vi "getData_v4.vi"() -> ()   [LabVIEW 2014]
uses:
  <vilib>/FPGAPlugInAG/cRIO-9039/niLvFpga_Open_cRIO-9039.vi
  <vilib>/Utility/error.llb/Error Cluster From Error Code.vi
  <vilib>/rvi/errors/niLvFpgaAdjustHostInterfaceError.vi
  <vilib>/Utility/file.llb/Write To Spreadsheet File (DBL).vi
  <vilib>/FPGAPlugInAG/cRIO-9039/niLvFpga_Close_cRIO-9039.vi
  <vilib>/rvi/interface/nirviOpenFPGA/nirviOpenFPGA.xnode
  FPGA Bitfiles/test0304_FPGATarget_imptestv12p4_nHMFqqsr4pc.lvbitx
  FPGA VIs/imp_test_v12_p4.vi
  <vilib>/rvi/interface/nirviMethod/nirviMethod.xnode
  <vilib>/rvi/interface/nirviCloseFPGA/nirviCloseFPGA.xnode
  <vilib>/FPGAPlugInAG/cRIO-9039/niLvFpga_ReadFifo_cRIO-9039.vi
  <vilib>/rvi/errors/niLvFpgaMergeErrorWithErrorCode.vi
panel:
  out "Timer (Sec)":u32
  out "FIFO empty":bool
  out "Elements Remaining":u32=10000
  in  "Time_read":i32=10000
  out "message":string=" INSTRUCTIONS:\r\rNormal Use:  When using subVIs that incorporate the error in/error out (or error I/O) structure, place this handler where you want to inform the user of an error, typically at the end of the I/O data path, as the last action of the program.  If the error in error? is ERROR, the handler creates a message describing the error and its source.  If the type of dialog = 1 (default), the message is displayed to the user, who can only acknowedge it.  If the type = 2, the user can acknowledge the message or abort execution; aborting a program with active I/O is not recommended.  If the type = 0, no message is displayed; this is used to process the error programmatically, and the error out cluster elements are wired to individual terminals for that reason.  \r\rOther Use:\n\r\nlocal testing.  To test the error code of a subVI or function that does not have the error I/O structure, you can wire its error code and a source string to the local error code and error source inputs.  If error in error? indicates no error and error code is not equal to 0, the local code and source are substituted for the error in values, and error? is set TRUE (ERROR)."
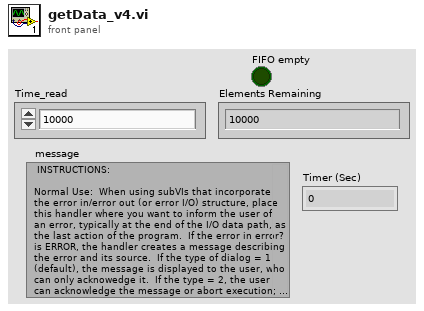
[diagram p1: front panel]
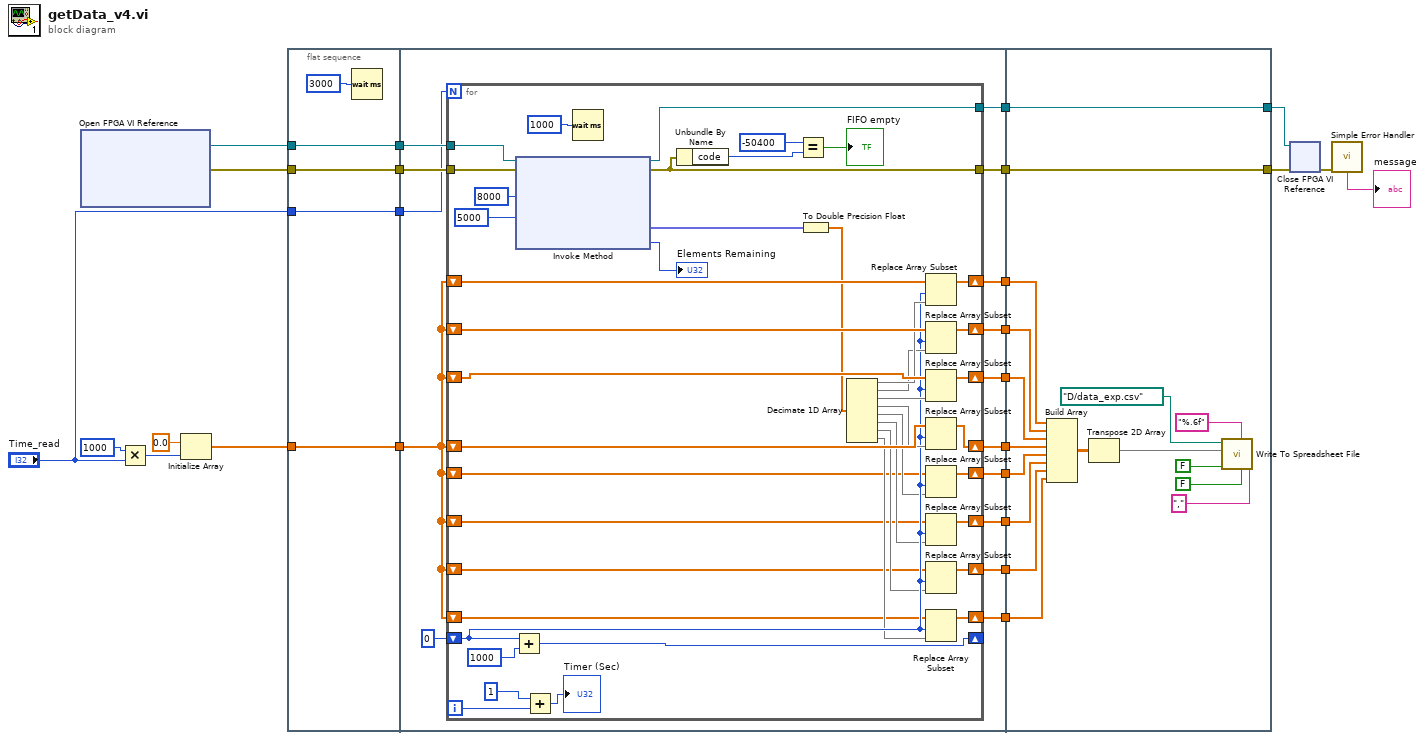
[diagram p0: block diagram]
diagram:
  n1 = xnode "Open FPGA VI Reference"() -> ("FPGA VI Reference Out"=w1:refnum<k20>, "error out"=w2:errorcluster)  [unwired: 2 in]
  n2 = Multiply(x=1000 ("y"), y="Time_read") -> (x*y=w18:i32)
  n3 = Initialize Array(0.0 ("element"), w18) -> (w22:dbl[])
  n4 = flat-sequence {
    tunnel: "Time_read" -> [w27]
    tunnel: w2 -> [w28]
    tunnel: w1 -> [w29]
    tunnel: w22 -> [w30]
    tunnel: [w30] -> w6
    tunnel: [w29] -> w5
    tunnel: [w28] -> w4
    tunnel: [w27] -> w3
    tunnel: [w42] -> w16
    tunnel: [w41] -> w15
    tunnel: [w40] -> w14
    tunnel: [w39] -> w13
    tunnel: [w38] -> w12
    tunnel: [w36] -> w11
    tunnel: [w35] -> w10
    tunnel: [w34] -> w9
    tunnel: [w33] -> w8
    tunnel: [w32] -> w7
    tunnel: w6 -> [w37]
    tunnel: w5 -> [w44]
    tunnel: w4 -> [w43]
    tunnel: w3 -> [w31]
    tunnel: w16 -> [w102]
    tunnel: w15 -> [w101]
    tunnel: w14 -> [w100]
    tunnel: [w105] -> w21
    tunnel: w13 -> [w105]
    tunnel: [w104] -> w20
    tunnel: w12 -> [w104]
    tunnel: w11 -> [w99]
    tunnel: w10 -> [w98]
    tunnel: w9 -> [w96]
    tunnel: w8 -> [w97]
    tunnel: w7 -> [w103]
    frame #0 {
      n5 = Wait (ms)(milliseconds to wait=u32 3000 ("y")) -> ()  [unwired: 1 out]
    }
    frame #1 {
      n6 = for {
        N: w31 -> [_]
        shift-right: [w86] -> _
        shift-left: 0 -> [w72]
        shift-right: [w75] -> w42
        shift-left: w37 -> [w84]
        shift-right: [w74] -> w41
        shift-left: w37 -> [w83]
        shift-right: [w73] -> w40
        shift-left: w37 -> [w82]
        shift-right: [w76] -> w32
        shift-left: w37 -> [w85]
        tunnel: w44 -> [w56]
        tunnel: w43 -> [w55]
        tunnel: [w51] -> w39
        tunnel: [w52] -> w38
        shift-right: [w66] -> w36
        shift-left: w37 -> [w67]
        shift-right: [w64] -> w35
        shift-left: w37 -> [w65]
        shift-right: [w63] -> w33
        shift-left: w37 -> [w62]
        shift-right: [w60] -> w34
        shift-left: w37 -> [w61]
        i -> [w48]
        n7 = Add(x=w72, y=1000) -> (x+y=w86:i32)
        n8 = xnode "Invoke Method"("FPGA VI Reference In"=w56, "error in"=w55, "Number of Elements"=u32 8000, "Timeout (ms)"=5000) -> ("FPGA VI Reference Out"=w51:refnum<k20>, "error out"=w52:errorcluster, "Data"=w49:fxp<+/-,46,20>[], "Elements Remaining"=→"Elements Remaining":u32)
        n9 = Add(x=1, y=w48) -> (x+y=→"Timer (Sec)":i32)
        n10 = Wait (ms)(milliseconds to wait=u32 1000 ("y")) -> ()  [unwired: 1 out]
        n11 = Unbundle By Name(w52) -> ("code"=w58:i32)
        n12 = Equal?(x=-50400 ("y"), y=w58) -> (x = y?=→"FIFO empty":bool)
        n13 = To Double Precision Float(number=w49) -> (double precision float=w81:dbl[])
        n14 = Decimate 1D Array(w81) -> (w80:dbl[], w79:dbl[], w78:dbl[], w77:dbl[], w71:dbl[], w70:dbl[], w69:dbl[], w68:dbl[])
        n15 = Replace Array Subset(array=w85, new element=w80, index=w72) -> (w76:dbl[])
        n16 = Replace Array Subset(array=w84, new element=w79, index=w72) -> (w75:dbl[])
        n17 = Replace Array Subset(array=w83, new element=w78, index=w72) -> (w74:dbl[])
        n18 = Replace Array Subset(array=w82, new element=w77, index=w72) -> (w73:dbl[])
        n19 = Replace Array Subset(array=w67, new element=w71, index=w72) -> (w66:dbl[])
        n20 = Replace Array Subset(array=w65, new element=w70, index=w72) -> (w64:dbl[])
        n21 = Replace Array Subset(array=w62, new element=w69, index=w72) -> (w63:dbl[])
        n22 = Replace Array Subset(array=w61, new element=w68, index=w72) -> (w60:dbl[])
      }
    }
    frame #2 {
      n23 = Build Array(w103, w102, w101, w100, w99, w98, w97, w96) -> (w89:dbl[][])
      n24 = Transpose 2D Array(2D array=w89) -> (transposed array=w94:dbl[][])
      n25 = call-poly <vilib>:"Write To Spreadsheet File.vi"("delimiter (\\t)"="," ("delimiter (\\t)"), "transpose? (no:F)"=FALSE, "format (%.3f)"="%.6f" ("format (%d)"), "append to file? (new file:F)"=FALSE, "2D data"=w94, "file path (dialog if empty)"=path "D:/data_exp.csv") -> ()  [unwired: 2 in, 1 out]
    }
  }
  n26 = xnode "Close FPGA VI Reference"("FPGA VI Reference In"=w21, "error in"=w20) -> ("error out"=w24:errorcluster)
  n27 = call <vilib>:"Simple Error Handler.vi"("error in (no error)"=w24) -> ("message"=→"message":string)  [unwired: 4 in, 4 out]
